vi "查询MN号.vi"(8 "error in (no error)":errorcluster caption="错误输入（无错误）", 11 "簇":cluster{"MN":string, "PW":string}={"MN"="平台数据发送系统", "PW"="平台数据发送系统"}) -> (0 "error out":errorcluster caption="错误输出", 3 "包含启动项":bool)   [LabVIEW 2016, in "数据传输系统-06.lvlib"]
uses:
  <vilib>/registry/registry.llb/Registry RtKey.ctl
  <vilib>/registry/registry.llb/Read Registry Value Simple STR.vi
panel:
  out "值":string[](array[string])
  out "名称":string[](array[string])
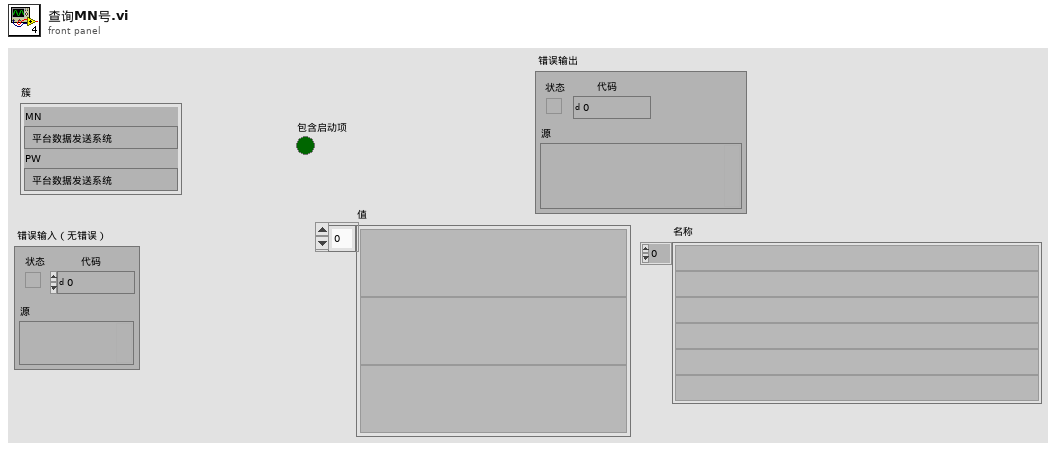
[diagram p1: front panel]
types:
  T1 = typedef "Registry RtKey.ctl" = enum32{"HKEY_CLASSES_ROOT", "HKEY_CURRENT_USER", "HKEY_LOCAL_MACHINE", "HKEY_USERS", "HKEY_PERFORMANCE_DATA", "HKEY_CURRENT_CONFIG", "HKEY_DYN_DATA"}
  T2 = typedef "Registry refnum.ctl" = refnum<k1>
  T3 = cluster{"numValues":i32, "maxValueNameLen":i32, "maxValueDataLen":i32}
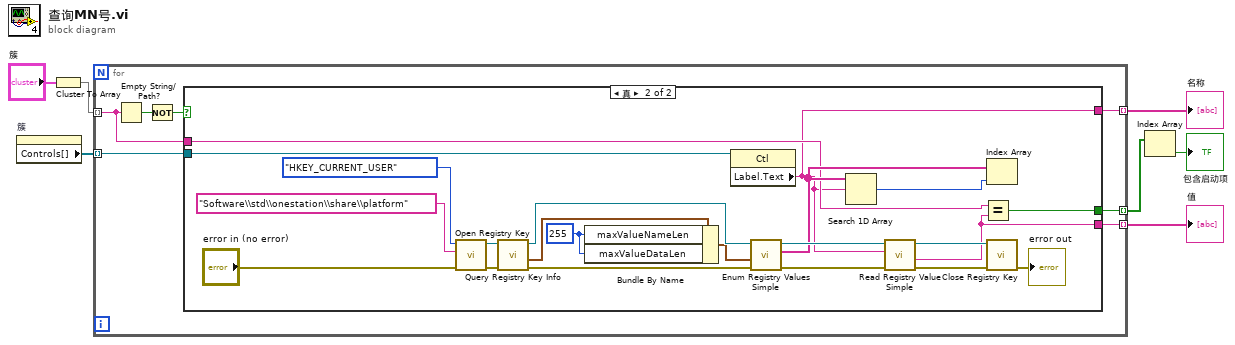
[diagram p0: block diagram]
diagram:
  n1 = property on="簇" class="Clust (严格)"() -> ("Controls[]"=w5:refnum<vi>[])  [unwired: 2 in, 2 out]
  n2 = Cluster To Array(cluster="簇") -> (array=w6:string[])
  n3 = for {
    tunnel: w6 -> [w12] mode=indexing
    tunnel: w5 -> [w11] mode=indexing
    tunnel: [w10] -> w4 mode=indexing
    tunnel: [w9] -> w2 mode=indexing
    tunnel: [w8] -> w3 mode=indexing
    n4 = Empty String/Path?(string/path=w12) -> (empty?=w14:bool)
    n5 = Not(x=w14) -> (.not. x?=w13:bool)
    n6 = case shown="真" w13 {
      tunnel: [_ w23] -> w9
      tunnel: w12 -> [_ w16]
      tunnel: w11 -> [_ w19]
      tunnel: [_ w18] -> w10
      tunnel: [_ w15] -> w8
      frame False {
      }
      frame True {
        w20 = 255 ("maxValueNameLen")
        n7 = call <vilib>:"Open Registry Key.vi"("error in (no error)"="error in (no error)", "subkey"="Software\\std\\onestation\\share\\platform", "root key (HKEY_LOCAL_MACHINE)"=Registry_RtKey."HKEY_CURRENT_USER") -> ("error out"=w33:errorcluster, "refnum out"=w34:T2)  [unwired: 7 in]
        n8 = call <vilib>:"Query Registry Key Info.vi"("error in (no error)"=w33, "refnum"=w34) -> ("error out"=w29:errorcluster, "value info"=w22:T3, "refnum out"=w30:T2)  [unwired: 5 in, 2 out]
        n9 = Bundle By Name(cluster=w22, "maxValueNameLen"=w20, "maxValueDataLen"=w20) -> (w21:T3)
        n10 = property class="Ctl"(reference=w19) -> ("Label.Text"=w15:string)  [unwired: 1 in, 2 out]
        n11 = call <vilib>:"Enum Registry Values Simple.vi"("error in (no error)"=w29, "value info"=w21, "refnum"=w30) -> ("error out"=w26:errorcluster, "values"=w17:string[], "refnum out"=w28:T2)  [unwired: 3 in, 3 out]
        n12 = Search 1D Array(1D array=w17, element=w15) -> (index of element=w24:i32)  [unwired: 1 in]
        n13 = call-poly <vilib>:"Read Registry Value Simple.vi"("error in (no error)"=w26, "value"=w15, "refnum"=w28) -> ("error out"=w25:errorcluster, "String/Binary data"=w18:string, "refnum out"=w27:T2)  [unwired: 3 in, 1 out]
        n14 = Equal?(x=w16, y=w18) -> (x = y?=w23:bool)
        n15 = Index Array(array=w17, index=w24) -> ()  [unwired: 1 out]
        n16 = call <vilib>:"Close Registry Key.vi"("error in (no error)"=w25, "refnum"=w27) -> ("error out"=→"error out":errorcluster)  [unwired: 5 in]
      }
    }
  }
  "值" <- w4
  "名称" <- w3
  n17 = Index Array(array=w2) -> (element=→"包含启动项":bool)  [unwired: 1 in]
